vi "Create Request-Reply.vi"(8 "error in (no error)":errorcluster, 11 "API-Reference in":refnum<data-value>) -> (0 "error out":errorcluster, 3 "API-Reference out":refnum<data-value>)   [LabVIEW 2018]
uses:
  Actor.lvclass
  Stopped.ctl
  Did Initialize.ctl
  Stop.ctl
  Message-Enqueuer References.ctl
  API-Data.ctl
  Launch.ctl
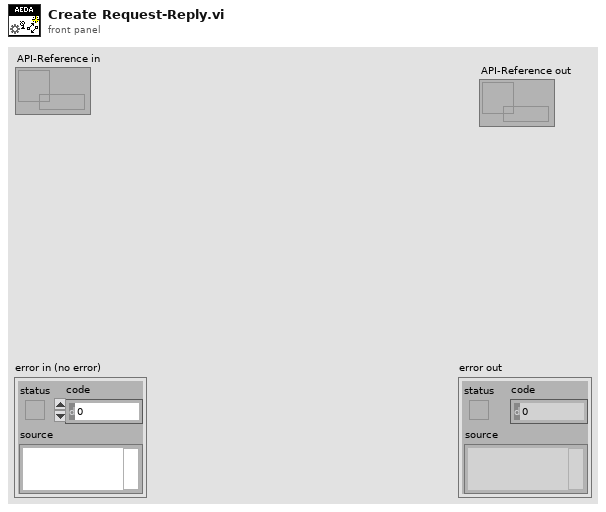
[diagram p1: front panel]
types:
  T1 = typedef "Actor.lvclass/API-Data.ctl" = cluster{"Launch":refnum<notifier>, "Did Stop Enqueuer":refnum<user-event>, "Message Enqueuers":T2, "Stopped Reg":refnum<event-registration>}
  T2 = typedef "Actor.lvclass/Message-Enqueuer References.ctl" = cluster{"Stop":refnum<user-event>, "Launch":refnum<user-event>, "Did Initialize":refnum<user-event>}
  T3 = typedef "Actor.lvclass/Stopped.ctl" = cluster{"State":refnum<class "Actor.lvclass">, "Final Error":errorcluster}
  T4 = cluster{"Stop":refnum<user-event>, cluster{"Stopped":refnum<user-event>, void}}
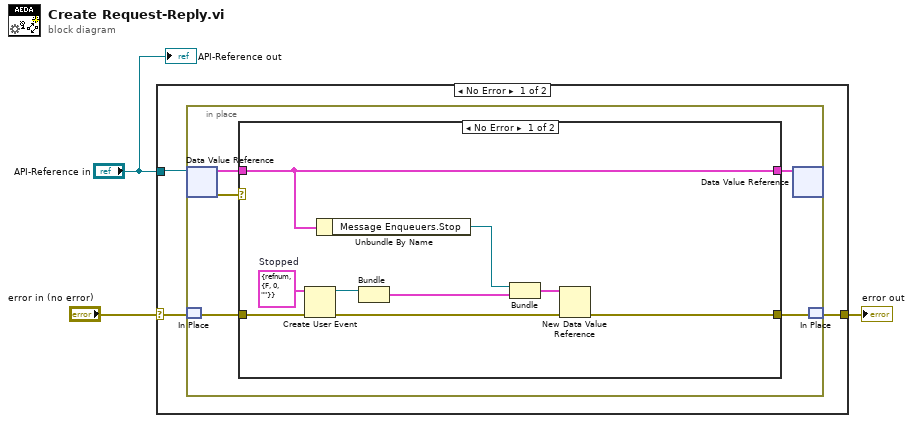
[diagram p0: block diagram]
diagram:
  n1 = case shown="No Error" "error in (no error)" {
    selector: "error in (no error)" -> [w6 w23]
    tunnel: [w5 w23] -> w2
    tunnel: "API-Reference in" -> [w4 _]
    frame No Error {
      n2 = in-place {
        n3 = in-place-dvr #1(w4) -> (w10:T1, w11:errorcluster)
        n4 = in-place-match #2(w6) -> (w8:errorcluster)
        n5 = case shown="No Error" w11 {
          selector: w11 -> [_ w22]
          tunnel: w10 -> [w20 w21]
          tunnel: [w20 w21] -> w9
          tunnel: w8 -> [w19 _]
          tunnel: [w15 w22] -> w7
          frame No Error {
            w12 = T3 {"State"=refnum, "Final Error"={"status"=FALSE, "code"=0, "source"=""}}  # Stopped
            n6 = Create User Event(user event datatype=w12, error in=w19) -> (user event=w14:refnum<user-event>, error out=w16:errorcluster)
            n7 = Unbundle By Name(w20) -> ("Message Enqueuers.Stop"=w13:refnum<user-event>)
            n8 = Bundle("Stopped"=w14) -> (w18:cluster{"Stopped":refnum<user-event>, void})  [unwired: 2 in]
            n9 = Bundle("Stop"=w13, w18) -> (w17:T4)  [unwired: 1 in]
            n10 = New Data Value Reference(data value=w17, error in=w16) -> (error out=w15:errorcluster)  [unwired: 1 out]
          }
          frame Error {
          }
        }
        n11 = in-place-dvr #1(w9) -> ()  [unwired: 2 out]
        n12 = in-place-match #2(w7) -> (w5:errorcluster)
      }
    }
    frame Error {
    }
  }
  "error out" <- w2
  "API-Reference out" <- "API-Reference in"
